vi "Generate control system simulated cycle.vi"(9 "ROI Dwell time (us)":dbl=4.0 min=0.05 max=20.0 step=0.05, 10 "Control system time resolution (0.05us)":dbl=0.05, 11 "Number of POI":i32=3) -> (1 "Time-stamps (us)":dbl[](array[numeric]) format="%.2f", 3 "Simulated control timings sequence (with Ref frames)":waveform(dbl)(graph))   [LabVIEW 2017]
panel:
  out "Number of timestamp indexes":i32
  out "Simulated control timings sequence (without Ref frames)":waveform(dbl)(graph)
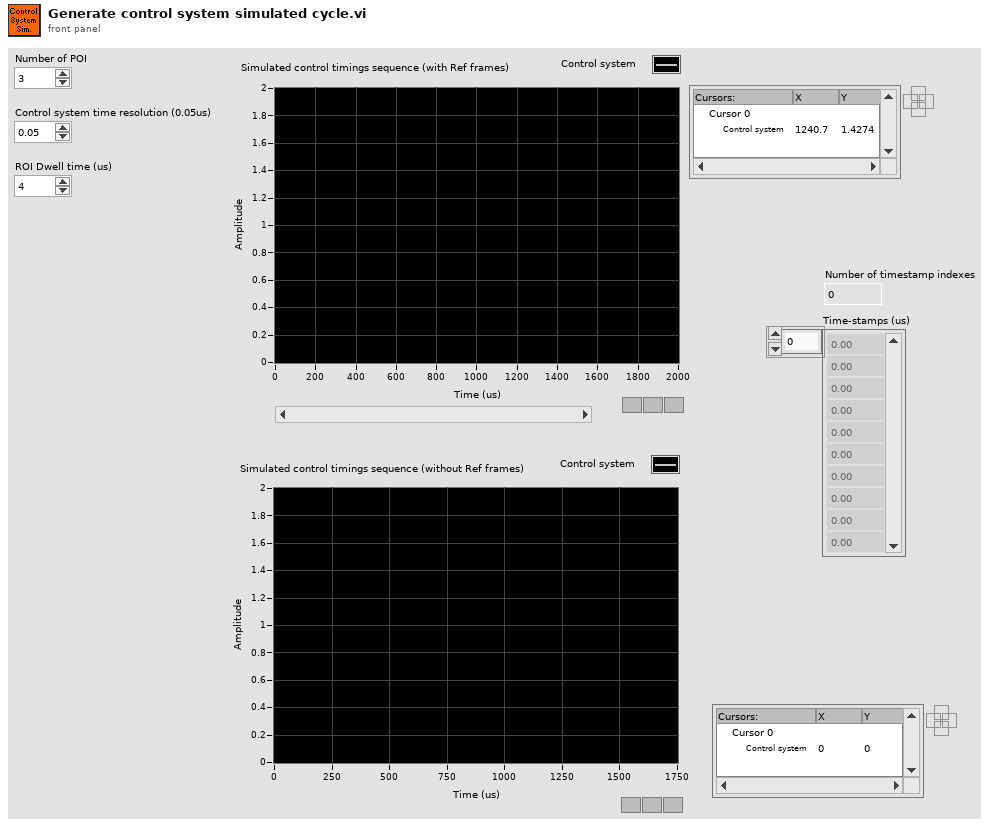
[diagram p1: front panel]
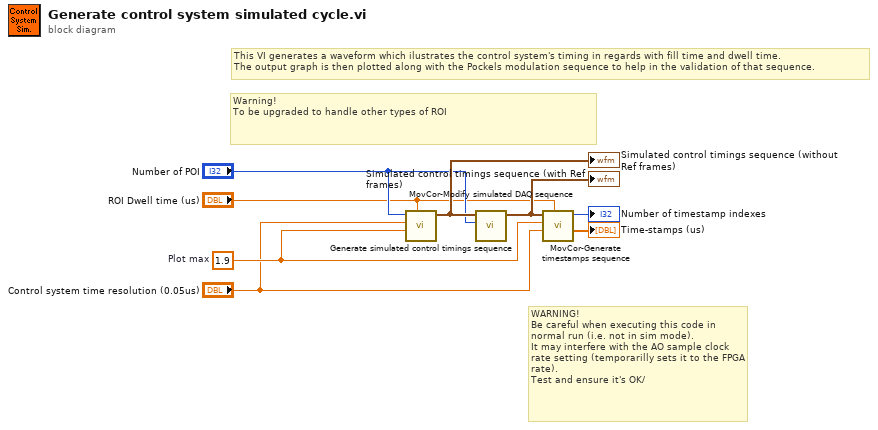
[diagram p0: block diagram]
diagram:
  w3 = 1.9  # Plot max
  # "WARNING!\nBe careful when executing this code in  normal run (i.e. not in sim mode). \nIt may interfere with the AO sample clock rate setting (temporarilly sets it to the FPGA rate).\nTest and ensure it's OK/"
  # "This VI generates a waveform which ilustrates the control system's timing in regards with fill time and dwell time.\nThe output graph is then plotted along with the Pockels modulation sequence to help in the validation of that sequence."
  # "Warning!\nTo be upgraded to handle other types of ROI"
  n1 = call "Generate simulated control timings sequence.vi"("ROI Dwell time"="ROI Dwell time (us)", "High value of simulated waveform"=w3, "Time resolution of simulated waveform"="Control system time resolution (0.05us)", "Number of POI"="Number of POI") -> ("Simulated control timings sequence in"=w5:waveform(dbl))  [unwired: 7 in]
  "Simulated control timings sequence (without Ref frames)" <- w5
  n2 = call "MovCor-Modify simulated DAQ sequence.vi"("Number of POI"="Number of POI", "Simulated control timings sequence in"=w5) -> ("Simulated control timings sequence"=w8:waveform(dbl))  [unwired: 9 in]
  "Simulated control timings sequence (with Ref frames)" <- w8
  n3 = call "MovCor-Generate timestamps sequence.vi"("ROI Dwell time (us)"="ROI Dwell time (us)", "Time resolution of simulated waveform"="Control system time resolution (0.05us)", "High value of simulated waveform"=w3, "Acquisition system simulated waveform"=w8) -> ("Time-stamps (us)"=→"Time-stamps (us)":dbl[], "Number of timestamp indexes"=→"Number of timestamp indexes":i32)  [unwired: 6 in]
